vi "AutoPush.vi"(7 "PushMode":T2, 8 "Max Power Out":dbl, 9 "MaxRPM":dbl, 10 "RPM":dbl, 11 "MotorIn":dbl) -> (3 "MotorOut":dbl)   [LabVIEW 2013]
uses:
  PushMode.ctl
  SingleSolenoidAction.ctl
  <vilib>/addons/control/pid/pid.llb/PID (DBL).vi
  <vilib>/addons/control/pid/NI_PID_pid.lvlib
panel:
  in  "PID gains":T1={"proportional gain (Kc)"=1.0, "integral time (Ti, min)"=0.01, "derivative time (Td, min)"=0.0} {"derivative time (Td, min)" format="%.3f"; "integral time (Ti, min)" format="%.3f"; "proportional gain (Kc)" format="%.3f"}
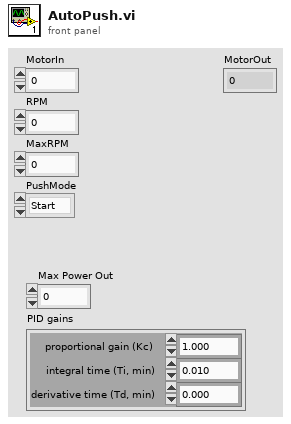
[diagram p1: front panel]
types:
  T1 = cluster{"proportional gain (Kc)":dbl, "integral time (Ti, min)":dbl, "derivative time (Td, min)":dbl}
  T2 = typedef "PushMode.ctl" = enum16{"Start", "Adjust", "Stop"}
  T3 = typedef "SingleSolenoidAction.ctl" = enum16{"Init", "SetState", "Disable"}
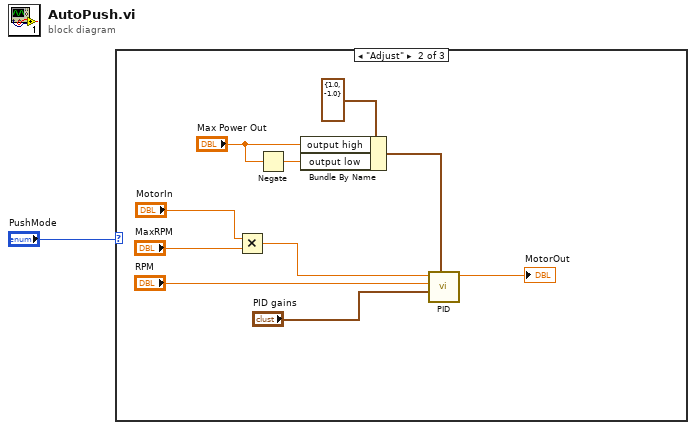
[diagram p0: block diagram]
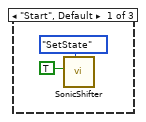
[diagram p2: hidden frame]
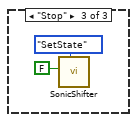
[diagram p3: hidden frame]
diagram:
  n1 = case shown="\"Adjust\"" "PushMode" {
    frame "Start", Default {
      n2 = call "SonicShifter.vi"("Action"=SingleSolenoidAction."SetState" ("Mode"), "Actuate?"=TRUE) -> ()  [unwired: 9 in, 1 out]
    }
    frame "Adjust" {
      n3 = Multiply(x="MotorIn", y="MaxRPM") -> (x*y=w9:dbl)
      n4 = Negate(x="Max Power Out") -> (-x=w6:dbl)
      n5 = Bundle By Name(cluster=cluster{"output high":dbl, "output low":dbl} {"output high"=1.0, "output low"=-1.0} ("output range"), "output high"="Max Power Out", "output low"=w6) -> (w5:cluster{"output high":dbl, "output low":dbl})
      n6 = call-poly <vilib>:"PID.vi"("output range"=w5, "PID gains"="PID gains", "process variable"="RPM", "setpoint"=w9) -> ("output"=→"MotorOut":dbl)  [unwired: 6 in, 1 out]
    }
    frame "Stop" {
      n7 = call "SonicShifter.vi"("Action"=SingleSolenoidAction."SetState" ("Mode"), "Actuate?"=FALSE) -> ()  [unwired: 9 in, 1 out]
    }
  }
